vi "_Axis_Rel.vi"(8 "Error In":errorcluster, 10 "相对位置":i32, 11 "轴序号":u16) -> (0 "Error Out":errorcluster)   [LabVIEW 2020, in "MT_API.lvlib"]
doc: "MT_API INT32 __stdcall MT_Set_Axis_Position_P_Target_Rel(WORD AObj,INT32 Value);"
uses:
  MT_API.lvlib
  MT_API_64.dll
panel:
  out "函数返回值":i32
  # "将轴移动到相对位置"
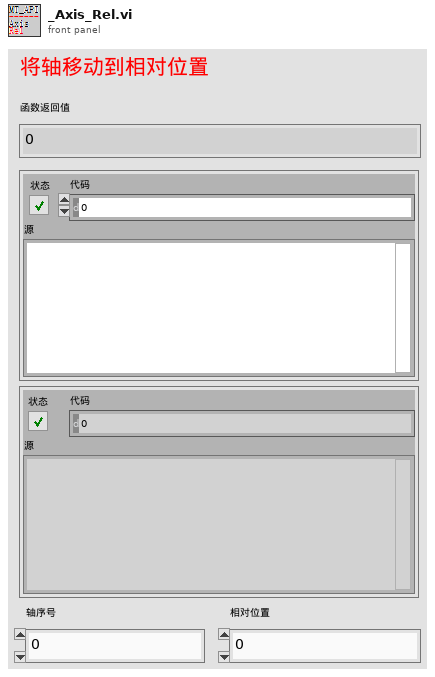
[diagram p1: front panel]
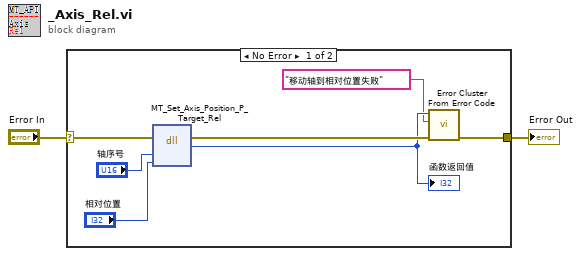
[diagram p0: block diagram]
diagram:
  n1 = case shown="No Error" "Error In" {
    selector: "Error In" -> [w9 w10]
    tunnel: [w7 w10] -> w1
    frame No Error {
      n2 = dll-call lib="D:/Project NJU/lib/MT/MT_API_64.*" fn="MT_Set_Axis_Position_P_Target_Rel"(error in=w9, "AObj"="轴序号", "Value"="相对位置") -> (error out=w8:errorcluster, "return type"=w4:i32)  [unwired: 4 in, 1 out]
      "函数返回值" <- w4
      n3 = call <vilib>:"Error Cluster From Error Code.vi"("error in (no error)"=w8, "error message (\"\")"="移动轴到相对位置失败", "error code (0)"=w4) -> ("error out"=w7:errorcluster)  [unwired: 6 in]
    }
    frame Error {
    }
  }
  "Error Out" <- w1
